vi "Chain.vi"(10 "Order":i32, 11 "Node to children":T2(c390)) -> (3 "Node to Order-Length Paths":T1(c390))   [LabVIEW 2024]
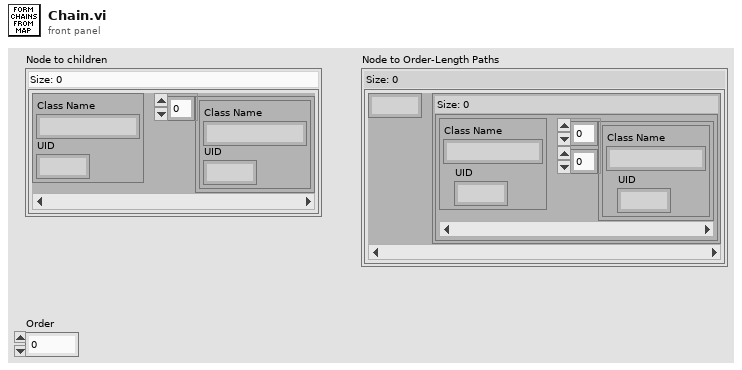
[diagram p1: front panel]
types:
  T1 = map{i32, map{cluster{"Class Name":string, "UID":i32}, cluster{"Class Name":string, "UID":i32}[][]}}
  T2 = map{cluster{"Class Name":string, "UID":i32}, cluster{"Class Name":string, "UID":i32}[]}
  T3 = map{cluster{"Class Name":string, "UID":i32}, cluster{"Class Name":string, "UID":i32}[][]}
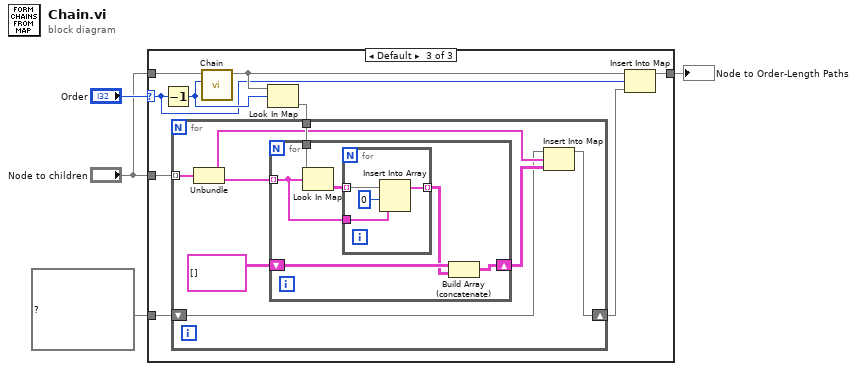
[diagram p0: block diagram]
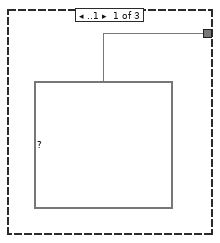
[diagram p2: hidden frame]
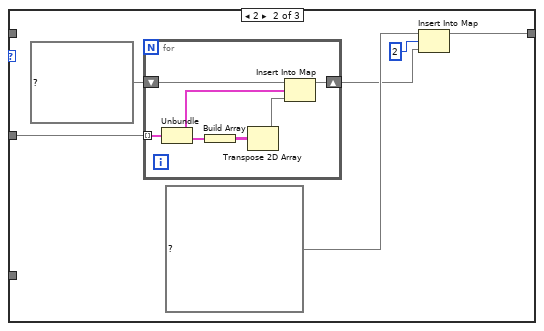
[diagram p3: hidden frame]
diagram:
  n1 = case shown="Default" "Order" {
    selector: "Order" -> [_ _ w19]
    tunnel: "Node to children" -> [_ _ w27]
    tunnel: "Node to children" -> [_ w10 w26]
    tunnel: T3 {} ("map in") -> [_ _ w25]
    tunnel: [T1 {} ("map") w6 w20] -> w1
    frame ..1 {
    }
    frame 2 {
      n2 = for {
        tunnel: w10 -> [w18] mode=indexing
        shift-right: [w14] -> w7
        shift-left: T3 {} ("map") -> [w17]
        n3 = Unbundle(w18) -> ("Source"=w16:cluster{"Class Name":string, "UID":i32}, "value"=w15:cluster{"Class Name":string, "UID":i32}[])
        n4 = Build Array(w15) -> (w13:cluster{"Class Name":string, "UID":i32}[][])
        n5 = Transpose 2D Array(2D array=w13) -> (transposed array=w12:cluster{"Class Name":string, "UID":i32}[][])
        n6 = Insert Into Map(map in=w17, key=w16, value=w12) -> (map out=w14:T3)  [unwired: 2 out]
      }
      n7 = Insert Into Map(map in=T1 {} ("map"), key=2, value=w7) -> (map out=w6:T1)  [unwired: 2 out]
    }
    frame Default {
      n8 = Decrement(x=w19) -> (x-1=w22:i32)
      n9 = call "Chain.vi"("Order"=w22, "Node to children"=w27) -> ("Node to Order-Length Paths"=w23:T1)  [unwired: 9 in]
      n10 = Look In Map(map=w23, key=w22) -> (value=w24:T3)  [unwired: 1 in, 1 out]
      n11 = for {
        tunnel: w24 -> [w33]
        tunnel: w26 -> [w35] mode=indexing
        shift-right: [w28] -> w21
        shift-left: w25 -> [w29]
        n12 = Unbundle(w35) -> ("Source"=w32:cluster{"Class Name":string, "UID":i32}, "value"=w34:cluster{"Class Name":string, "UID":i32}[])
        n13 = for {
          tunnel: w34 -> [w39] mode=indexing
          tunnel: w33 -> [w41]
          shift-right: [w37] -> w30
          shift-left: cluster{"Class Name":string, "UID":i32}[][] [] ("value") -> [w38]
          n14 = Look In Map(map=w41, key=w39) -> (value=w40:cluster{"Class Name":string, "UID":i32}[][])  [unwired: 1 in, 1 out]
          n15 = for {
            tunnel: w40 -> [w45] mode=indexing
            tunnel: w39 -> [w43]
            tunnel: [w42] -> w36 mode=indexing
            n16 = Insert Into Array(array=w45, index=0, new element=w43) -> (w42:cluster{"Class Name":string, "UID":i32}[])
          }
          n17 = Build Array (concatenate)(w38, w36) -> (w37:cluster{"Class Name":string, "UID":i32}[][])
        }
        n18 = Insert Into Map(map in=w29, key=w32, value=w30) -> (map out=w28:T3)  [unwired: 2 out]
      }
      n19 = Insert Into Map(map in=w23, key=w19, value=w21) -> (map out=w20:T1)  [unwired: 2 out]
    }
  }
  "Node to Order-Length Paths" <- w1
